vi "CLD 15 Parsing SubVI.vi"(8 "Error In":errorcluster, 11 "all rows in":string[][](array[string])) -> (0 "Error Out":errorcluster, 3 "Data Out":T1[](array[typedef]))   [LabVIEW 2009]
doc: "CLD 15 This SubVI parses the array data into the format required by the specification for CLD 15. There are multiple ways to approach the decoding of the string data. \n\nCase 0 uses fixed location of the digits and Case 1 uses regular expressions to separate text and 'numbers' within the data string.\n\nThe data format from the specification is pasted as a free label for programming convenience."
uses:
  CLD 15 CSV file data structure.ctl
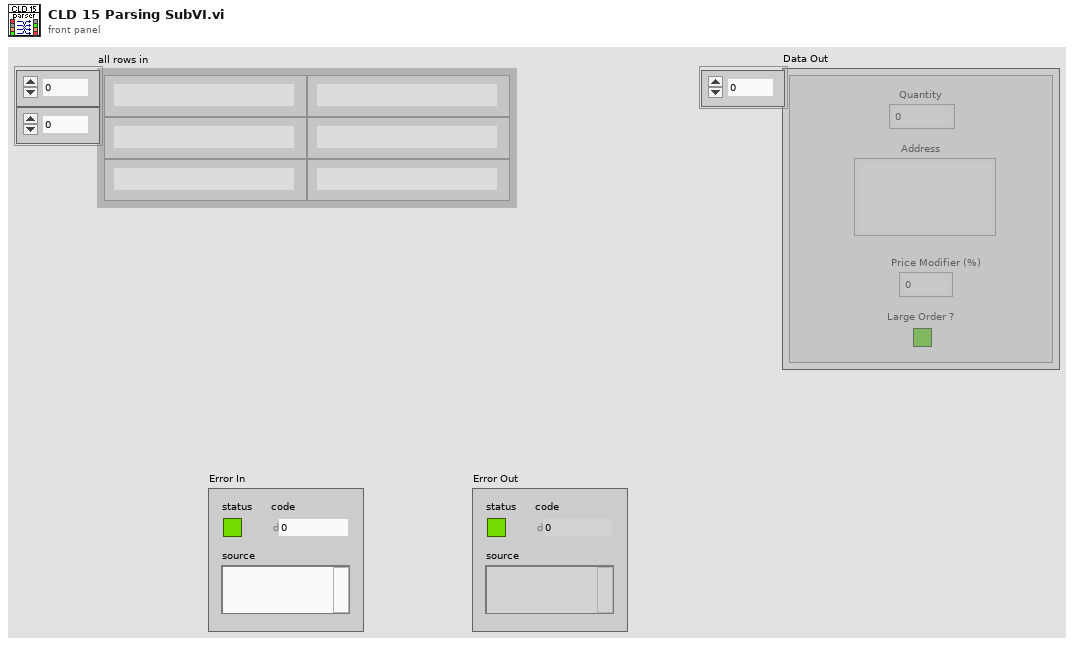
[diagram p1: front panel]
types:
  T1 = typedef "CLD 15 CSV file data structure.ctl" = cluster{"Quantity":i32, "Address":string, "Price Modifier (%)":dbl, "Large Order ?":bool}
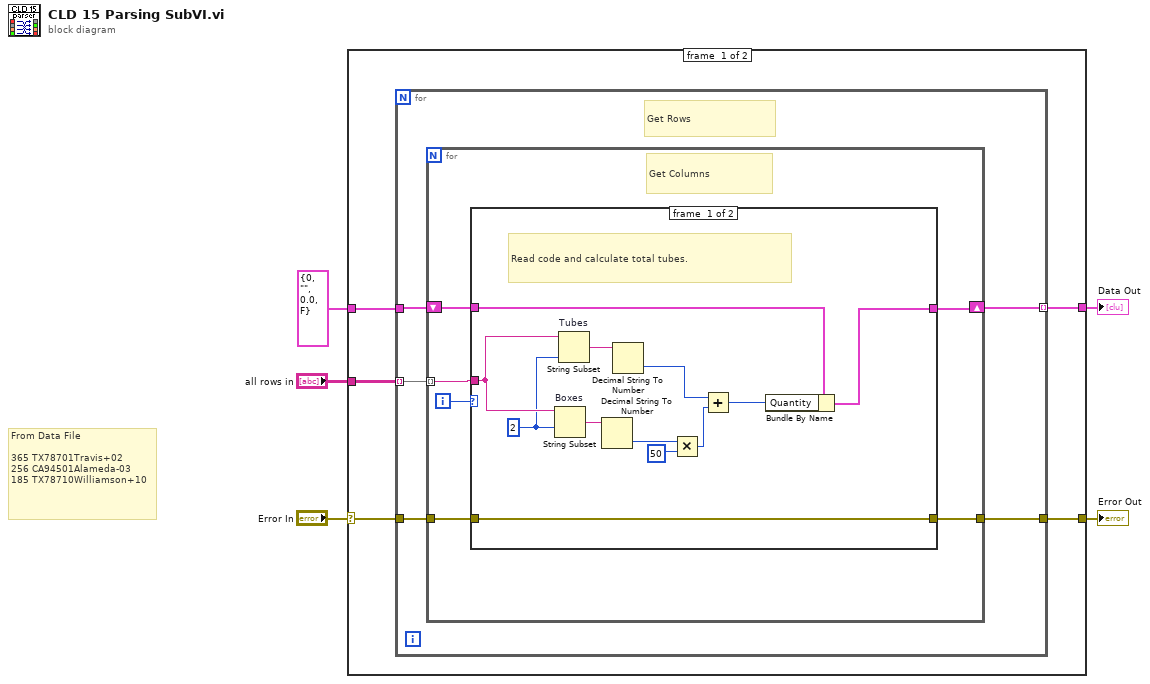
[diagram p0: block diagram]
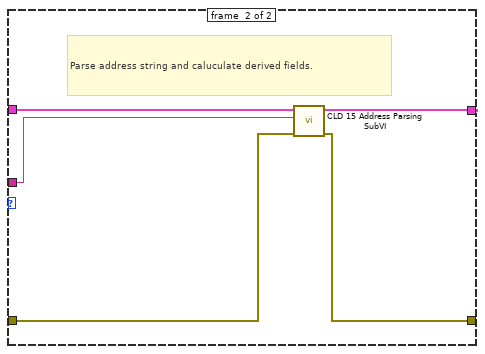
[diagram p2: hidden frame]
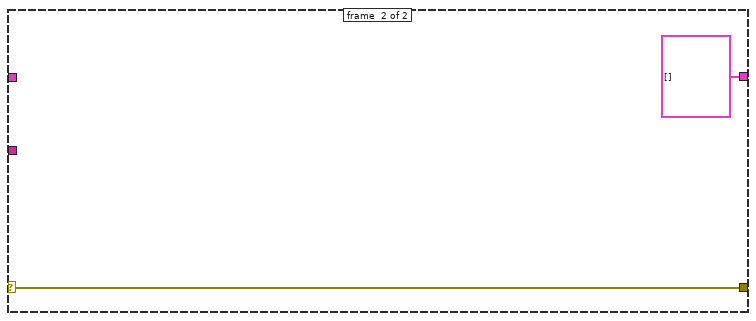
[diagram p3: hidden frame]
diagram:
  # "From Data File\n\n365\tTX78701Travis+02\n256\tCA94501Alameda-03\n185\tTX78710Williamson+10"
  n1 = case shown="No Error" "Error In" {
    selector: "Error In" -> [w7 w39]
    tunnel: [w10 w39] -> w5
    tunnel: T1 {"Quantity"=0, "Address"="", "Price Modifier (%)"=0.0, "Large Order ?"=FALSE} ("CSV File Data Structure") -> [w9 _]
    tunnel: [w8 T1[] []] -> w3
    tunnel: "all rows in" -> [w6 _]
    frame #0 {
      n2 = for {
        tunnel: w7 -> [w15]
        tunnel: [w14] -> w10
        tunnel: w9 -> [w13]
        tunnel: [w12] -> w8 mode=indexing
        tunnel: w6 -> [w11] mode=indexing
        # "Get Rows"
        n3 = for {
          tunnel: w15 -> [w18]
          tunnel: [w17] -> w14
          shift-right: [w19] -> w12
          shift-left: w13 -> [w20]
          tunnel: w11 -> [w16] mode=indexing
          i -> [w21]
          # "Get Columns"
          n4 = case shown="1" w21 {
            tunnel: w16 -> [w33 w38]
            tunnel: w20 -> [w30 w37]
            tunnel: [w29 w36] -> w19
            tunnel: w18 -> [w22 w35]
            tunnel: [w22 w34] -> w17
            frame #0 {
              w23 = 2 ("length (rest)")
              # "Read code and calculate total tubes."
              n5 = String Subset "Boxes"(string=w33, offset (0)=w23) -> (substring=w31:string)  [unwired: 1 in]
              n6 = String Subset "Tubes"(string=w33, length (rest)=w23) -> (substring=w32:string)  [unwired: 1 in]
              n7 = Decimal String To Number(string=w31) -> (number=w27:i32)  [unwired: 2 in, 1 out]
              n8 = Decimal String To Number(string=w32) -> (number=w28:i32)  [unwired: 2 in, 1 out]
              n9 = Multiply(x=w27, y=50) -> (x*y=w24:i32)
              n10 = Add(x=w28, y=w24) -> (x+y=w25:i32)
              n11 = Bundle By Name(cluster=w30, "Quantity"=w25) -> (w29:T1)
            }
            frame #1 {
              # "Parse address string and caluculate derived fields."
              n12 = call "CLD 15 Address Parsing SubVI.vi"("error in"=w35, "Data String in"=w38, "CSV File Data Structure in"=w37) -> ("error out"=w34:errorcluster, "CSV File Data Structure out"=w36:T1)  [unwired: 7 in]
            }
          }
        }
      }
    }
    frame #1 {
    }
  }
  "Error Out" <- w5
  "Data Out" <- w3
